vi "Configure Inhibit Input.vi"(8 "error in (no error)":errorcluster, 10 "Inhibit Input (2: Off)":i32(ring)=2 items=["Latching", "Live", "Off"], 11 "VISA resource name":refnum<visa-resource-name>) -> (0 "error out":errorcluster, 3 "VISA resource name out":refnum<visa-resource-name>)   [LabVIEW 2020, in "Keysight E36300 Series.lvlib"]
doc: "Configures the operation mode of the inhibit input.\n\n<b>Note: </b>\nThis VI is only available on the E36312A and E36313A models."
uses:
  Keysight E36300 Series.lvlib
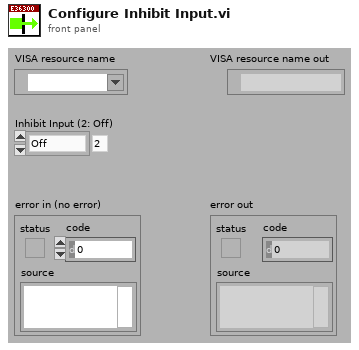
[diagram p1: front panel]
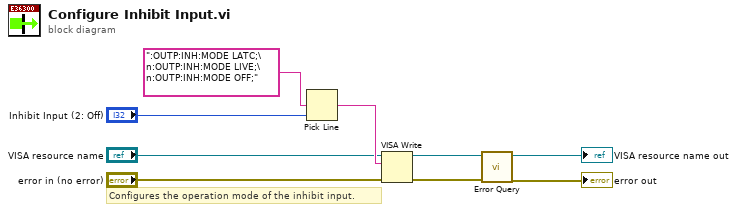
[diagram p0: block diagram]
diagram:
  # "Configures the operation mode of the inhibit input."
  n1 = Pick Line(multi-line string=":OUTP:INH:MODE LATC;\n:OUTP:INH:MODE LIVE;\n:OUTP:INH:MODE OFF;", line index="Inhibit Input (2: Off)") -> (output string=w7:string)  [unwired: 1 in]
  n2 = VISA Write(VISA resource name="VISA resource name", write buffer=w7, error in (no error)="error in (no error)") -> (VISA resource name out=w4:refnum<visa-resource-name>, error out=w3:errorcluster)  [unwired: 1 out]
  n3 = call "Error Query.vi"("error in (no error)"=w3, "VISA resource name"=w4) -> ("error out"=→"error out":errorcluster, "VISA resource name out"=→"VISA resource name out":refnum<visa-resource-name>)  [unwired: 6 in, 2 out]
